vi "Ascenseur.vi"   [LabVIEW 2018]
uses:
  MyGlobal.vi
  <vilib>/addons/control/pid/pid.llb/PID (DBL).vi
  <vilib>/addons/control/pid/NI_PID_pid.lvlib
types:
  T1 = cluster{"proportional gain (Kc)":dbl, "integral time (Ti, min)":dbl, "derivative time (Td, min)":dbl}
  T2 = typedef "WPI_PotentiometerDevRef.ctl" = cluster{"DevStatus":errorcluster, "Analog Channel":T3, "Invert Output":bool}
  T3 = typedef "FPGA_AIChannel.ctl" = enum8{"AI 0", "AI 1", "AI 2", "AI 3", "AI MXP 0", "AI MXP 1", "AI MXP 2", "AI MXP 3", "Invalid"}
  T4 = typedef "WPI_MotorControlDeviceRef.ctl" = cluster{"DeviceStatus":errorcluster, "Type":T5, "PWM":cluster{"PWM Channel":T6, "DeadBand":T7}, "CAN":cluster{"Device Number":u8, "SetOutput VI Ref":variant, "GetOutput VI Ref":variant, "Enable VI Ref":variant, "Disable VI Ref":variant, "Data":variant}, "Invert":bool, "DIO PWM":cluster{"PWM \"Enable\" Channel":T6, "DIOChannel":T8, "PWM Rate":dbl}}
  T5 = typedef "WPI_MotorControlType.ctl" = enum16{"PWM", "CAN", "DIO PWM"}
  T6 = typedef "FPGA_DIOPWMChannel.ctl" = enum8{"PWM 0", "PWM 1", "PWM 2", "PWM 3", "PWM 4", "PWM 5", "PWM 6", "PWM 7", "PWM 8", "PWM 9", "PWM MXP 0", "PWM MXP 1", "PWM MXP 2", "PWM MXP 3", "PWM MXP 4", "PWM MXP 5", "PWM MXP 6", "PWM MXP 7", "PWM MXP 8", "PWM MXP 9", "Invalid"}
  T7 = typedef "WPI_PWMDeadband.ctl" = cluster{"Name":string, "maxPositivePwm":i32, "minPositivePwm":i32, "centerPwm":i32, "maxNegativePwm":i32, "minNegativePwm":i32, "angularRange":u16}
  T8 = typedef "FPGA_DIOChannel.ctl" = enum8{"DIO 0", "DIO 1", "DIO 2", "DIO 3", "DIO 4", "DIO 5", "DIO 6", "DIO 7", "DIO 8", "DIO 9", "DIO MXP 0", "DIO MXP 1", "DIO MXP 2", "DIO MXP 3", "DIO MXP 4", "DIO MXP 5", "DIO MXP 6", "DIO MXP 7", "DIO MXP 8", "DIO MXP 9", "DIO MXP 10", "DIO MXP 11", "DIO MXP 12", "DIO MXP 13", "DIO MXP 14", "DIO MXP 15", "SPI Port CS1", "SPI Port CS2", "SPI Port CS3", "SPI Port MISO", "SPI Port MOSI", "Invalid"}
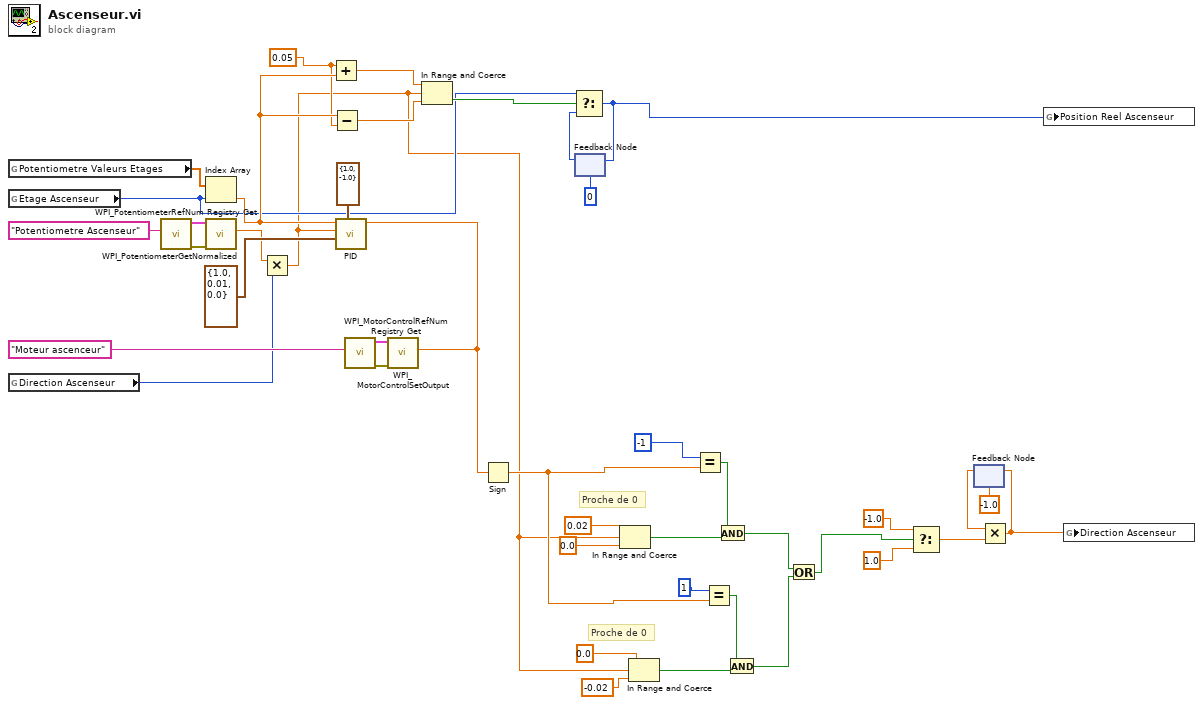
[diagram p0: block diagram]
diagram:
  w32 = 0.05
  # "Proche de 0"
  # "Proche de 0"
  n1 = global read "MyGlobal.vi" "Potentiometre Valeurs Etages"() -> (w34:dbl[])
  n2 = global read "MyGlobal.vi" "Etage Ascenseur"() -> (w28:u8)
  n3 = global read "MyGlobal.vi" "Direction Ascenseur"() -> (w12:u8)
  n4 = call <vilib>:"WPI_PotentiometerRefNum Registry Get.vi"("refnum name"="Potentiometre Ascenseur") -> ("error out"=w37:errorcluster, "PotDevRef"=w36:T2)  [unwired: 9 in]
  n5 = Index Array(array=w34, index=w28) -> (element=w33:dbl)
  n6 = call <vilib>:"WPI_PotentiometerGetNormalized.vi"("error in"=w37, "PotDevRef"=w36) -> ("Normalized Value"=w14:dbl)  [unwired: 7 in, 2 out]
  n7 = Multiply(x=w14, y=w12) -> (x*y=w4:dbl)
  n8 = Add(x=w32, y=w33) -> (x+y=w30:dbl)
  n9 = Subtract(x=w33, y=w32) -> (x-y=w31:dbl)
  n10 = call-poly <vilib>:"PID.vi"("output range"=cluster{"output high":dbl, "output low":dbl} {"output high"=1.0, "output low"=-1.0}, "PID gains"=T1 {"proportional gain (Kc)"=1.0, "integral time (Ti, min)"=0.01, "derivative time (Td, min)"=0.0}, "process variable"=w4, "setpoint"=w33) -> ("output"=w11:dbl)  [unwired: 6 in, 1 out]
  n11 = call <vilib>:"WPI_MotorControlRefNum Registry Get.vi"("refnum name"="Moteur ascenceur") -> ("error out"=w41:errorcluster, "MotorControlDevRef"=w40:T4)  [unwired: 9 in]
  n12 = call <vilib>:"WPI_MotorControlSetOutput.vi"("error in (no error)"=w41, "Output"=w11, "MotorControlDevRef"=w40) -> ()  [unwired: 6 in, 3 out]
  n13 = In Range and Coerce(upper limit=w30, x=w4, lower limit=w31) -> (In Range?=w29:bool)  [unwired: 1 out]
  n14 = Sign(1:w11) -> (0:w5:dbl)
  n15 = feedback #1(0) -> (w26:i32)
  n16 = Select(t=w28, s=w29, f=w26) -> (s? t:f=w27:i32)
  n17 = feedback-in #1(w27) -> ()
  n18 = In Range and Coerce(upper limit=0.02, x=w4, lower limit=0.0) -> (In Range?=w22:bool)  [unwired: 1 out]
  n19 = In Range and Coerce(upper limit=0.0, x=w4, lower limit=-0.02) -> (In Range?=w8:bool)  [unwired: 1 out]
  n20 = Equal?(x=-1, y=w5) -> (x = y?=w20:bool)
  n21 = Equal?(x=1, y=w5) -> (x = y?=w10:bool)
  n22 = And(x=w20, y=w22) -> (x .and. y?=w3:bool)
  n23 = And(x=w10, y=w8) -> (x .and. y?=w2:bool)
  n24 = Or(x=w3, y=w2) -> (x .or. y?=w1:bool)
  n25 = Select(t=-1.0, s=w1, f=1.0) -> (s? t:f=w17:dbl)
  n26 = feedback #2(-1.0) -> (w15:dbl)
  n27 = Multiply(x=w15, y=w17) -> (x*y=w13:dbl)
  n28 = feedback-in #2(w13) -> ()
  n29 = global write "MyGlobal.vi" "Position Reel Ascenseur"(w27) -> ()
  n30 = global write "MyGlobal.vi" "Direction Ascenseur"(w13) -> ()
